vi "SetPropValve.vi"(0 "FPGA API in":refnum<class "FPGA API Mock.lvclass">, 5 "AO 1":dbl, 11 "error in (no error)":errorcluster) -> (4 "FPGA API out":refnum<class "FPGA API Mock.lvclass">, 15 "error out":errorcluster)   [LabVIEW 2019, in "FPGA API Mock.lvclass"]
uses:
  FPGA API Mock.lvclass
  FPGA API Mock.lvclass/FPGA API Mock.ctl
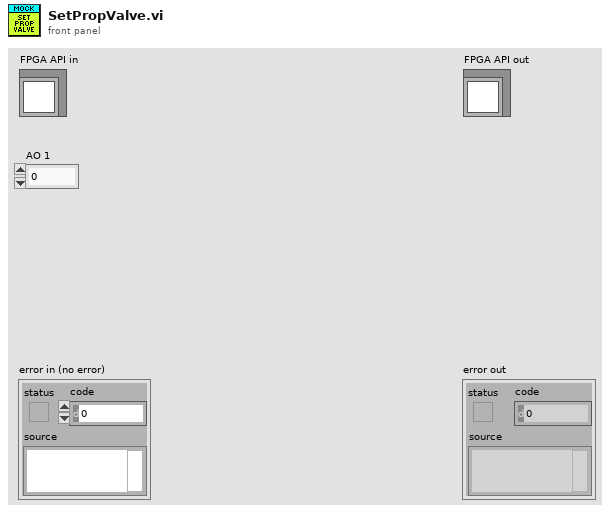
[diagram p1: front panel]
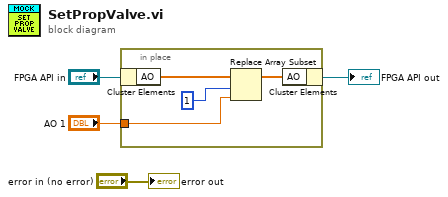
[diagram p0: block diagram]
diagram:
  n1 = in-place {
    in-place-border: "AO 1" -> [w5]
    n2 = in-place-cluster #1("FPGA API in") -> ("AO"=w8:dbl[])
    n3 = Replace Array Subset(array=w8, new element=w5, index=1) -> (w7:dbl[])
    n4 = in-place-cluster #1("AO"=w7) -> (→"FPGA API out":refnum<class "FPGA API Mock.lvclass">)
  }
  "error out" <- "error in (no error)"
